vi "Crop Image.vi"(11 "Camera Image":T1) -> (2 "Y Resolution":i32, 3 "Cropped Image":T1, 4 "X Resolution":i32)   [LabVIEW 2012]
uses:
  <vilib>/vision/Image Controls.llb/IMAQ Image.ctl
  <vilib>/vision/NI_Vision_Development_Module.lvlib
panel:
  in  "Botom Percent":dbl=0.45
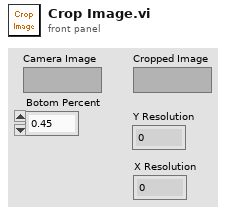
[diagram p1: front panel]
types:
  T1 = typedef "IMAQ Image.ctl" = refnum<image>
  T2 = typedef "Image Type" = u32
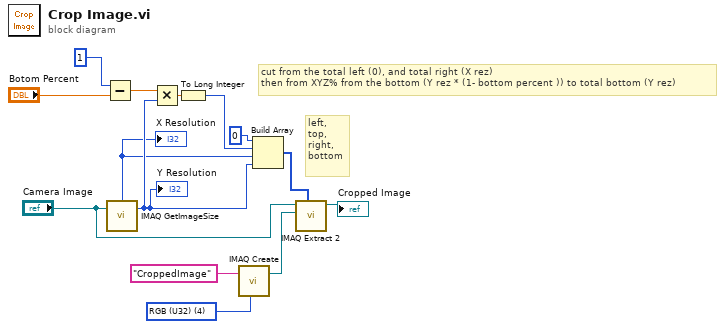
[diagram p0: block diagram]
diagram:
  w3 = T2 4 items=["Grayscale (U8)", "Grayscale (I16)", "Grayscale (SGL)", "Complex (CSG)", "RGB (U32)", "HSL (U32)", "RGB (U64)", "Grayscale (U16)"] ("Image Type")
  # "cut from the total left (0), and total right (X rez)\nthen from XYZ% from the bottom (Y rez * (1- bottom percent )) to total bottom (Y rez)"
  # "left, \ntop, \nright, \nbottom"
  n1 = Subtract(x=1, y="Botom Percent") -> (x-y=w11:dbl)
  n2 = call "IMAQ GetImageSize"("Image"="Camera Image") -> ("Y Resolution"=w2:i32, "X Resolution"=w1:i32)  [unwired: 3 in, 1 out]
  "Y Resolution" <- w2
  "X Resolution" <- w1
  n3 = Multiply(x=w11, y=w2) -> (x*y=w8:dbl)
  n4 = To Long Integer(number=w8) -> (32bit integer=w10:i32)
  n5 = call "IMAQ Create"("Image Name"="CroppedImage", "Image Type"=w3) -> ("New Image"=w5:T1)  [unwired: 3 in, 1 out]
  n6 = Build Array(0, w10, w1, w2) -> (w9:i32[])
  n7 = call "IMAQ Extract 2"("Optional Rectangle"=w9, "Image Dst"=w5, "Image Src"="Camera Image") -> ("Image Dst Out"=→"Cropped Image":T1)  [unwired: 7 in, 1 out]
